vi "get tcp ip server connection status.vi"(8 "error in (no error)":errorcluster, 11 "tcp ip server in":refnum<class "tcp ip server.lvclass">) -> (0 "error out":errorcluster, 2 "Connected?":bool, 3 "tcp ip server out":refnum<class "tcp ip server.lvclass">)   [LabVIEW 2020, in "tcp ip server.lvclass"]
uses:
  tcp ip server.lvclass
  tcp ip server.lvclass/tcp ip server.ctl
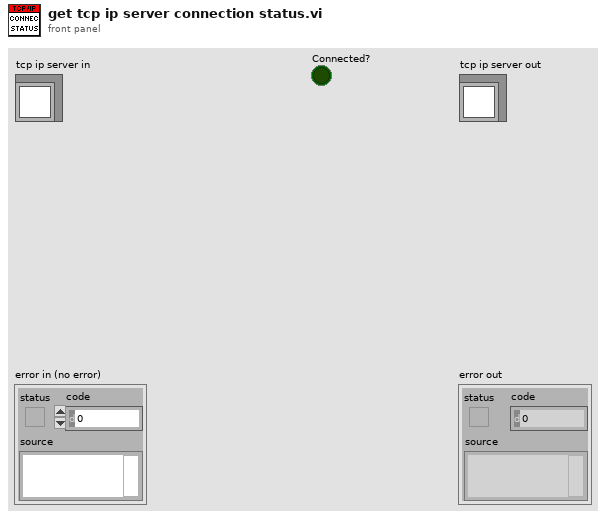
[diagram p1: front panel]
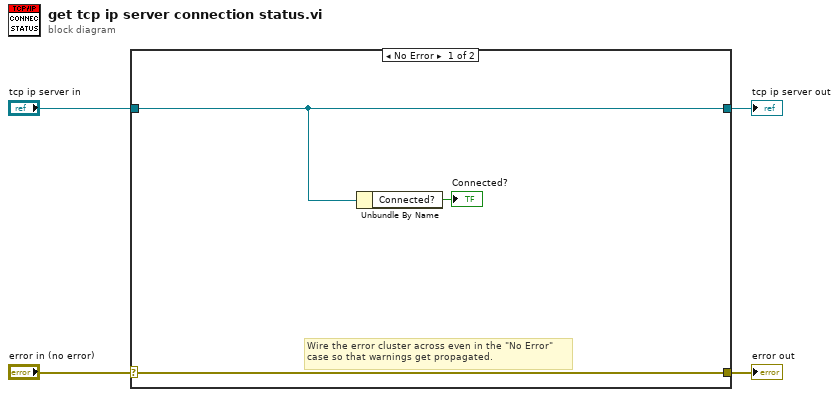
[diagram p0: block diagram]
diagram:
  n1 = case shown="No Error" "error in (no error)" {
    selector: "error in (no error)" -> [w7 w9]
    tunnel: [w7 w9] -> w3
    tunnel: [w6 w8] -> w1
    tunnel: "tcp ip server in" -> [w6 w8]
    frame No Error {
      # "Wire the error cluster across even in the \"No Error\"\ncase so that warnings get propagated."
      n2 = Unbundle By Name(w6) -> ("Connected?"=→"Connected?":bool)
    }
    frame Error {
    }
  }
  "error out" <- w3
  "tcp ip server out" <- w1
